vi "forceDemand.vi"(8 "error in (no error)":errorcluster, 9 "Force Demand":T1 min=-888.0 max=888.0 format="%.2f", 10 "model":refnum<class "Model.lvclass">, 11 "InteractiveMotionState in":refnum<class "InteractiveMotionState.lvclass">) -> (0 "error out":errorcluster, 2 "model 2":refnum<class "Model.lvclass">, 3 "InteractiveMotionState out":refnum<class "InteractiveMotionState.lvclass">)   [LabVIEW 2013, in "InteractiveMotionState.lvclass"]
uses:
  InteractiveMotionState.lvclass
  Model/Model/Model.lvclass
  Typedefs/ForceDemand.ctl
  Typedefs/FAMTTypedefs.lvlib
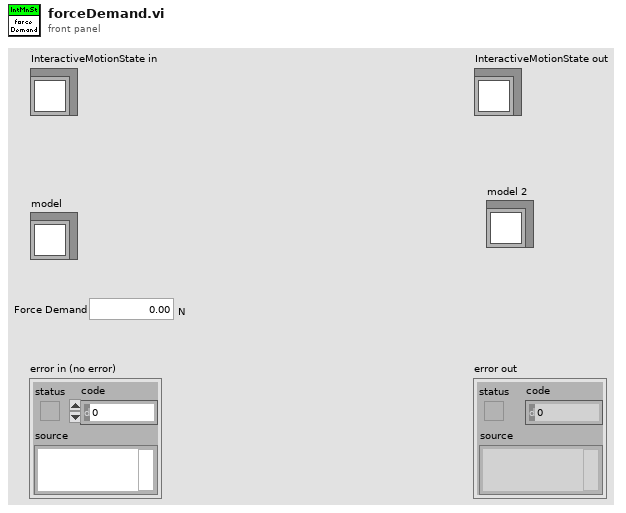
[diagram p1: front panel]
types:
  T1 = typedef "FAMTTypedefs.lvlib/ForceDemand.ctl" = dbl[unit]
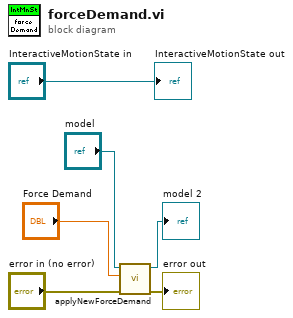
[diagram p0: block diagram]
diagram:
  n1 = call "applyNewForceDemand.vi"("error in (no error)"="error in (no error)", "Force Demand"="Force Demand", "Model in"="model") -> ("error out"=→"error out":errorcluster, "Model out"=→"model 2":refnum<class "Model.lvclass">)  [unwired: 7 in]
  "InteractiveMotionState out" <- "InteractiveMotionState in"
